vi "KE6221 -- PDelta Mode Get Params.vi"(0 "6221 Resource In":refnum<visa-resource-name>, 1 "Check For SCPI Errors? (T)":bool=TRUE, 11 "error in (no error)":errorcluster) -> (4 "6221 Resource Out (dupl)":refnum<visa-resource-name>, 8 "Pulsed Delta Mode Params":T1={"High Level (A)"=0.001, "Low Level (A)"=0.0, "Pulse Width (s)"=0.00011, "Source Delay (s)"=1.6e-05, "Num Cycles Mode"=enum."Finite Count", "Finite Count"=1, "Ranging Mode"=enum."Best", "Num Low Meas Per Cycle"=enum."1", "Pulse Period (Num PLCs)"=5, "Pulse Sweep Mode Enabled?"=FALSE} {"Pulse Period (Num PLCs)" min=5 max=999990; "Source Delay (s)" min=1.6e-05 max=0.011966 format="%.3p"; "Pulse Width (s)" min=5e-05 max=0.012 format="%.3p"; "Finite Count" min=1 max=65536; "Low Level (A)" min=-0.105 max=0.0 format="%.3p"; "High Level (A)" min=0.0 max=0.105 format="%.3p"}, 15 "error out":errorcluster)   [LabVIEW 2019, in "Keithley 622x.lvlib"]
doc: "Returns the parameters for 'Pulsed Delta' measurements. Note that 'Pulsed Delta' measurements are only available on the 6221, and performing this measurement implies that the 6221 is being used in conjuction with a 2182/2182A nano-voltmeter."
uses:
  Keithley 622x.lvlib
  Typedefs/KE6221 -- PDelta Mode Params.ctl
  Low Level/Typedefs/KE622x -- Delta PDelta Mode High Level.ctl
  Low Level/Typedefs/KE622x -- Delta PDelta Mode Low Level.ctl
  Low Level/Typedefs/KE6221 -- PDelta Mode Pulse Width.ctl
  Low Level/Typedefs/KE6221 -- PDelta Mode Source Delay.ctl
  Low Level/Typedefs/KE622x -- Delta PDelta Mode Num Cycles Mode.ctl
  Low Level/Typedefs/KE622x -- Delta PDelta Mode Num Cycles.ctl
  Low Level/Typedefs/KE6221 -- PDelta Mode Ranging Mode.ctl
  Low Level/Typedefs/KE6221 -- PDelta Mode Num Low Meas.ctl
  Low Level/Typedefs/KE6221 -- PDelta Mode Pulse Period.ctl
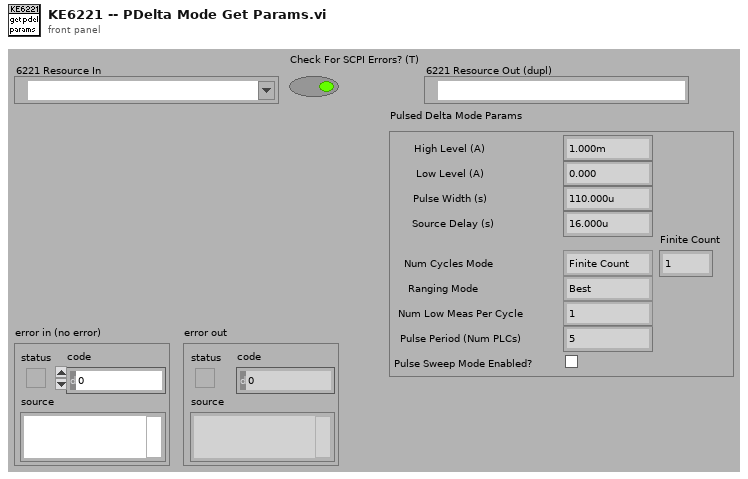
[diagram p1: front panel]
types:
  T1 = typedef "Keithley 622x.lvlib/KE6221 -- PDelta Mode Params.ctl" = cluster{"High Level (A)":T2, "Low Level (A)":T3, "Pulse Width (s)":T4, "Source Delay (s)":T5, "Num Cycles Mode":T6, "Finite Count":T7, "Ranging Mode":T8, "Num Low Meas Per Cycle":T9, "Pulse Period (Num PLCs)":T10, "Pulse Sweep Mode Enabled?":bool}
  T2 = typedef "Keithley 622x.lvlib/KE622x -- Delta PDelta Mode High Level.ctl" = dbl
  T3 = typedef "Keithley 622x.lvlib/KE622x -- Delta PDelta Mode Low Level.ctl" = dbl
  T4 = typedef "Keithley 622x.lvlib/KE6221 -- PDelta Mode Pulse Width.ctl" = dbl
  T5 = typedef "Keithley 622x.lvlib/KE6221 -- PDelta Mode Source Delay.ctl" = dbl
  T6 = typedef "Keithley 622x.lvlib/KE622x -- Delta PDelta Mode Num Cycles Mode.ctl" = enum16{"Finite Count", "Infinite"}
  T7 = typedef "Keithley 622x.lvlib/KE622x -- Delta PDelta Mode Num Cycles.ctl" = u32
  T8 = typedef "Keithley 622x.lvlib/KE6221 -- PDelta Mode Ranging Mode.ctl" = enum16{"Best", "Fixed"}
  T9 = typedef "Keithley 622x.lvlib/KE6221 -- PDelta Mode Num Low Meas.ctl" = enum16{"1", "2"}
  T10 = typedef "Keithley 622x.lvlib/KE6221 -- PDelta Mode Pulse Period.ctl" = u32
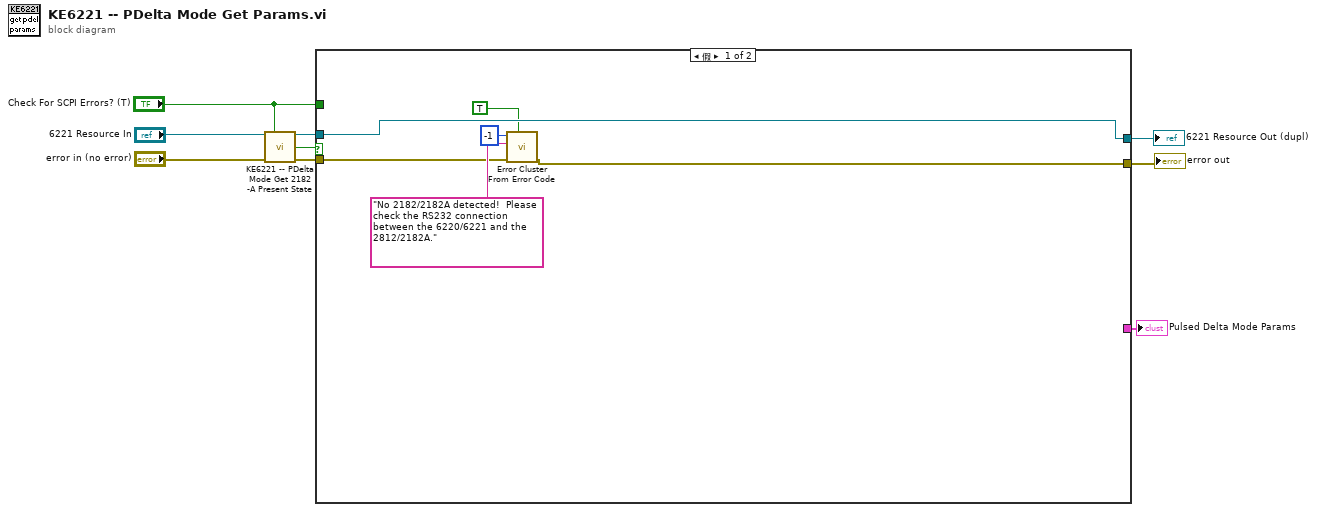
[diagram p0: block diagram]
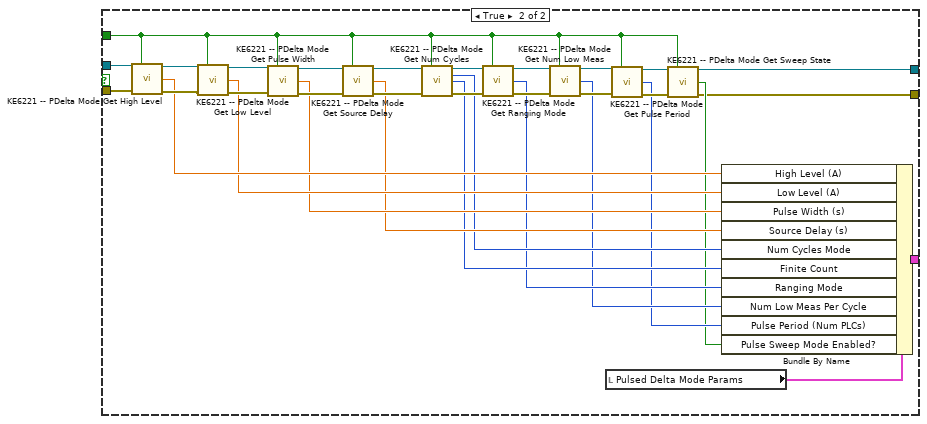
[diagram p2: hidden frame]
diagram:
  n1 = call "KE6221 -- PDelta Mode Get 2182 -A Present State.vi"("Resource In"="6221 Resource In", "Check For SCPI Errors? (T)"="Check For SCPI Errors? (T)", "error in (no error)"="error in (no error)") -> ("Resource Out (dupl)"=w8:refnum<visa-resource-name>, "2182/2182A Present?"=w1:bool, "error out"=w7:errorcluster)  [unwired: 10 in]
  n2 = case shown="假" w1 {
    tunnel: [_ w21] -> w9
    tunnel: w8 -> [w12 w20]
    tunnel: w7 -> [w13 w19]
    tunnel: "Check For SCPI Errors? (T)" -> [_ w18]
    tunnel: [w12 w17] -> w3
    tunnel: [w11 w16] -> w2
    frame False {
      n3 = call <vilib>:"Error Cluster From Error Code.vi"("show call chain? (False)"=TRUE, "error in (no error)"=w13, "error message (\"\")"="No 2182/2182A detected!  Please check the RS232 connection between the 6220/6221 and the 2812/2182A.", "error code (0)"=-1) -> ("error out"=w11:errorcluster)  [unwired: 5 in]
    }
    frame True {
      n4 = call "KE6221 -- PDelta Mode Get High Level.vi"("Resource In"=w20, "Check For SCPI Errors? (T)"=w18, "error in (no error)"=w19) -> ("Resource Out (dupl)"=w48:refnum<visa-resource-name>, "High Level (A)"=w31:T2, "error out"=w47:errorcluster)  [unwired: 10 in]
      n5 = call "KE6221 -- PDelta Mode Get Low Level.vi"("Resource In"=w48, "Check For SCPI Errors? (T)"=w18, "error in (no error)"=w47) -> ("Resource Out (dupl)"=w46:refnum<visa-resource-name>, "Low Level (A)"=w30:T3, "error out"=w45:errorcluster)  [unwired: 10 in]
      n6 = call "KE6221 -- PDelta Mode Get Pulse Width.vi"("Resource In"=w46, "Check For SCPI Errors? (T)"=w18, "error in (no error)"=w45) -> ("Resource Out (dupl)"=w44:refnum<visa-resource-name>, "Pulse Width (s)"=w29:T4, "error out"=w43:errorcluster)  [unwired: 10 in]
      n7 = call "KE6221 -- PDelta Mode Get Source Delay.vi"("Resource In"=w44, "Check For SCPI Errors? (T)"=w18, "error in (no error)"=w43) -> ("Resource Out (dupl)"=w40:refnum<visa-resource-name>, "Source Delay (s)"=w28:T5, "error out"=w39:errorcluster)  [unwired: 10 in]
      n8 = call "KE6221 -- PDelta Mode Get Num Cycles.vi"("Resource In"=w40, "Check For SCPI Errors? (T)"=w18, "error in (no error)"=w39) -> ("Resource Out (dupl)"=w42:refnum<visa-resource-name>, "Num Cycles Mode"=w27:T6, "Finite Count"=w26:T7, "error out"=w41:errorcluster)  [unwired: 9 in]
      n9 = call "KE6221 -- PDelta Mode Get Ranging Mode.vi"("Resource In"=w42, "Check For SCPI Errors? (T)"=w18, "error in (no error)"=w41) -> ("Resource Out (dupl)"=w36:refnum<visa-resource-name>, "Ranging Mode"=w25:T8, "error out"=w35:errorcluster)  [unwired: 10 in]
      n10 = call "KE6221 -- PDelta Mode Get Num Low Meas.vi"("Resource In"=w36, "Check For SCPI Errors? (T)"=w18, "error in (no error)"=w35) -> ("Resource Out (dupl)"=w34:refnum<visa-resource-name>, "Num Low Meas Per Cycle"=w24:T9, "error out"=w33:errorcluster)  [unwired: 10 in]
      n11 = local read "Pulsed Delta Mode Params"() -> (w32:T1)
      n12 = call "KE6221 -- PDelta Mode Get Pulse Period.vi"("Resource In"=w34, "Check For SCPI Errors? (T)"=w18, "error in (no error)"=w33) -> ("Resource Out (dupl)"=w38:refnum<visa-resource-name>, "Pulse Period (Num PLCs)"=w23:T10, "error out"=w37:errorcluster)  [unwired: 10 in]
      n13 = call "KE6221 -- PDelta Mode Get Sweep State.vi"("Resource In"=w38, "Check For SCPI Errors? (T)"=w18, "error in (no error)"=w37) -> ("Resource Out (dupl)"=w17:refnum<visa-resource-name>, "Sweep Enabled?"=w22:bool, "error out"=w16:errorcluster)  [unwired: 10 in]
      n14 = Bundle By Name(cluster=w32, "High Level (A)"=w31, "Low Level (A)"=w30, "Pulse Width (s)"=w29, "Source Delay (s)"=w28, "Num Cycles Mode"=w27, "Finite Count"=w26, "Ranging Mode"=w25, "Num Low Meas Per Cycle"=w24, "Pulse Period (Num PLCs)"=w23, "Pulse Sweep Mode Enabled?"=w22) -> (w21:T1)
    }
  }
  "Pulsed Delta Mode Params" <- w9
  "6221 Resource Out (dupl)" <- w3
  "error out" <- w2
